vi "document_wrapper.vi"(11 "BSONbytes":u8[](array[numeric])) -> (3 "BSONdoc":u8[](array[numeric]))   [LabVIEW 2015, in "BSON_convertors_Library.lvlib"]
doc: "Created by Artem Shevelev\nLabVIEW Portal profile: http://www.labviewportal.org/memberlist.php?mode=viewprofile&u=2340\ne-mail: artem.sh@gmail.com\nshevelev.pro"
uses:
  BSON_convertors_Library.lvlib
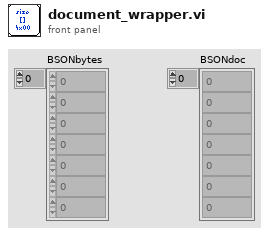
[diagram p1: front panel]
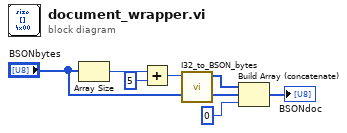
[diagram p0: block diagram]
diagram:
  n1 = Array Size(array="BSONbytes") -> (size(s)=w3:i32)
  n2 = Add(x=w3, y=5) -> (x+y=w5:i32)
  n3 = call "I32_to_BSON_bytes.vi"("value"=w5) -> ("BSONbytes"=w6:u8[])  [unwired: 10 in]
  n4 = Build Array (concatenate)(w6, "BSONbytes", u8 0 ("y")) -> (→"BSONdoc":u8[])
